vi "global-CSMQ FGV Change Flag.vi"() -> ()   [LabVIEW 2017, in "Communicable State Machine.lvlib"]
doc: "Global variable used to indicate whether the CSM module management information has changed"
uses:
  Communicable State Machine.lvlib
panel:
  in  "global-CSMQ FGV Change Flag":u64=4603270806574966694 format="%08x"
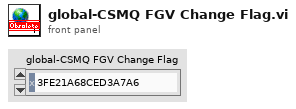
[diagram p1: front panel]
diagram:
